vi "dds_host.vi"() -> ()   [LabVIEW 2018]
uses:
  <vilib>/FPGAPlugInAG/PCIe-7841R/niLvFpga_Open_PCIe-7841R.vi
  <vilib>/rvi/interface/common/dynamic/niFpgaDynamicAddResources.vi
  <vilib>/FPGAPlugInAG/Dynamic/niLvFpga_Run_Dynamic.vi
  <vilib>/Utility/error.llb/Error Cluster From Error Code.vi
  <vilib>/rvi/errors/niLvFpgaAdjustHostInterfaceError.vi
  <vilib>/FPGAPlugInAG/Dynamic/niLvFpga_Close_Dynamic.vi
  <vilib>/rvi/interface/nirviOpenFPGA/nirviOpenFPGA.xnode
  FPGA Bitfiles/dds_FPGATarget_ddsfpga_kTR-VUpZgFc.lvbitx
  <vilib>/rvi/interface/nirviMethod/nirviMethod.xnode
  <vilib>/rvi/interface/nirviReadWriteControl/nirviReadWriteControl.xnode
  <vilib>/rvi/interface/nirviCloseFPGA/nirviCloseFPGA.xnode
  <vilib>/rvi/interface/Simulation/niFpgaSimulationCallBeginRW.vi
  NiFpgaLv.dll
  <vilib>/rvi/Analysis/host/Public/NI_FpgaMspHost.lvlib
panel:
  out "slow_freq":dbl
  out "scale factor_slow-dds":fxp<+/-,16,1>
  in  "vpp_slow-dds":dbl
  in  "slow-dds_param":T1={"Sine wave frequency (Hz)"=50.0, "Phase offset (deg)"=0.0} {"Phase offset (deg)" format="%#_6p"; "Sine wave frequency (Hz)" format="%#_6p"}
  in  "z_slow-dds?":bool
  in  "45_sin":bool=TRUE
  in  "23_sin":bool
  in  "01_sin":bool=TRUE
  in  "just x?":bool
  out "synth_settings_client":dbl[](array[numeric])=[8.0, 50000.0]
  out "scale factor 45":fxp<+/-,16,1>=0.20001220703125
  out "scale factor 23":fxp<+/-,16,1>=0.20001220703125
  out "scale factor 01":fxp<+/-,16,1>
  in  "set xy drive network?":bool
  in  "vpp 45":dbl=4.0
  in  "vpp 23":dbl=4.0
  in  "vpp 01":dbl
  in  "Desired loop rate (ticks)":u32=84
  in  "frequency increment":dbl=0.1
  out "requested_freq":dbl(graph)
  out "Sampling Rate\nAchieved?":bool=TRUE
  out "Actual Sample Rate (S/s)":dbl=952380.9523809524 format="%#_6p"
  in  "re-initialize_dds":bool
  in  "fast-dds_param":T1={"Sine wave frequency (Hz)"=50000.0, "Phase offset (deg)"=0.0} {"Phase offset (deg)" format="%#_6p"; "Sine wave frequency (Hz)" format="%#_6p"}
  in  "step_time (ms)":u32=1
  out "error out":errorcluster={"status"=TRUE, "code"=-61169, "source"="sample rate conversion in NI_FpgaMspHost.lvlib:Sample Rate To Loop Time (ticks).vi->dds_host.vi"}
  in  "stop":bool
  # "SINE"
  # "COSINE"
  # "SINE"
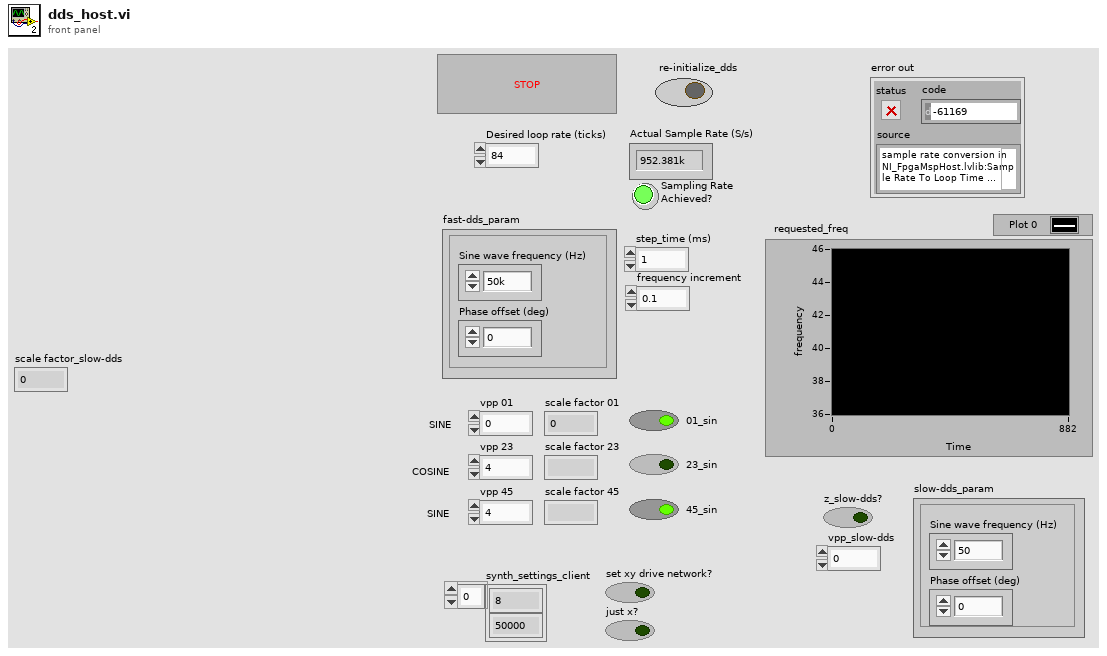
[diagram p1: front panel]
types:
  T1 = cluster{"Sine wave frequency (Hz)":dbl, "Phase offset (deg)":dbl}
  T2 = enum16{"open", "replace", "create", "open or create", "replace or create", "replace or create with confirmation"}
  T3 = cluster{"frequency (periods/tick)":fxp<+,32,0>, "phase offset (periods)":fxp<+,32,0>, fxp<+/-,16,1>, fxp<+,1,1>}
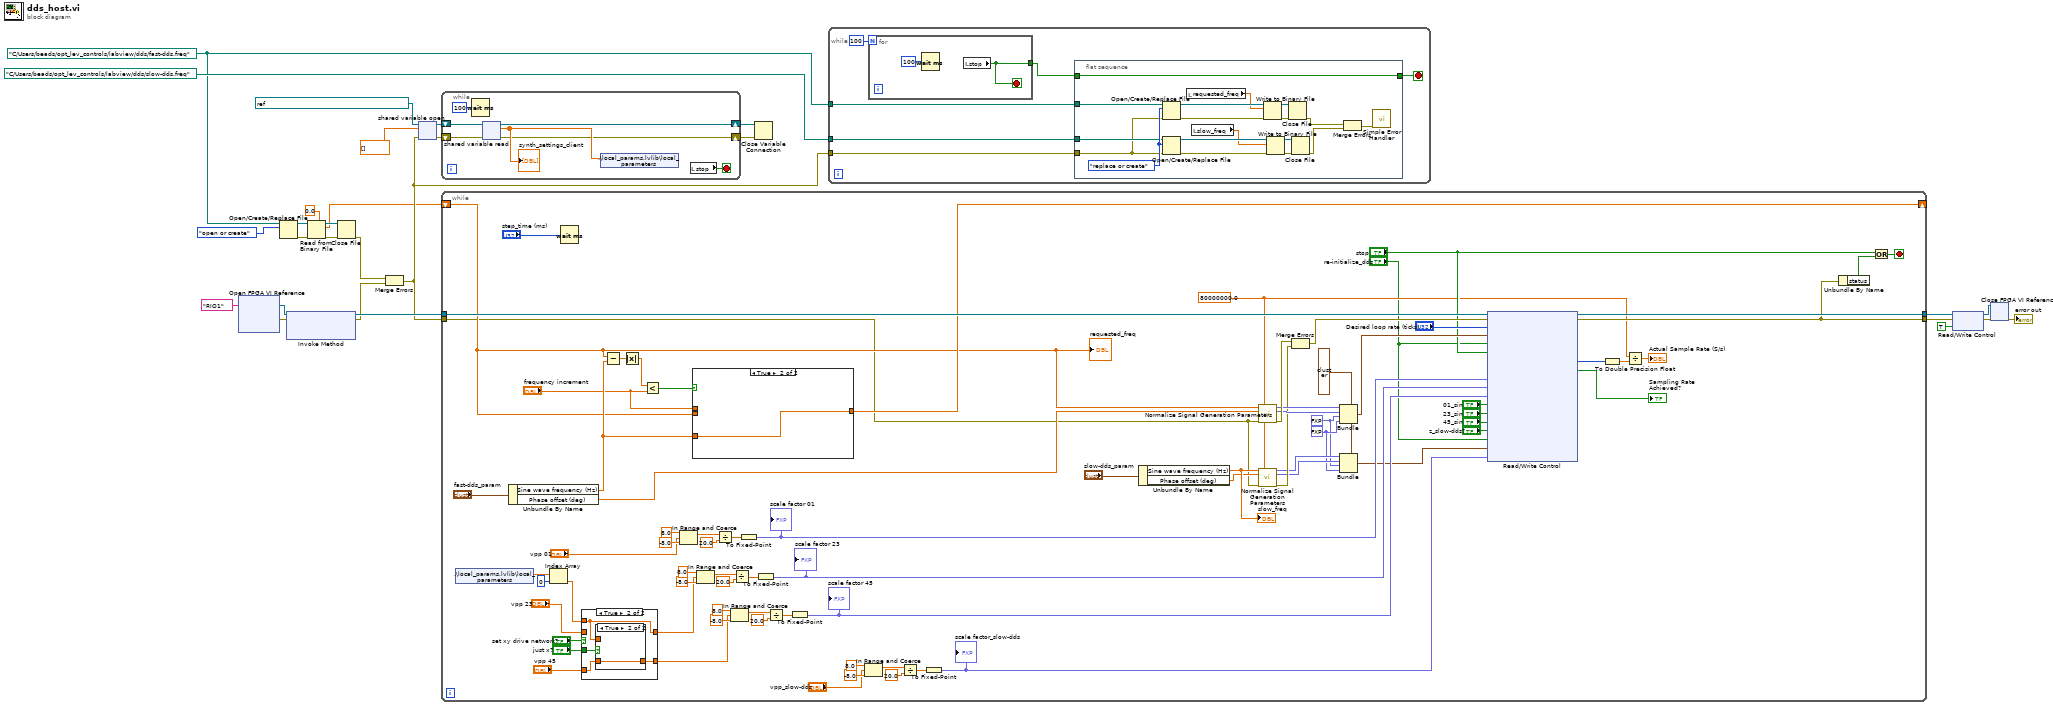
[diagram p0: block diagram]
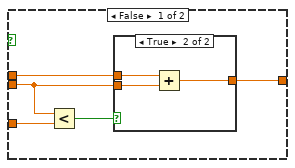
[diagram p4: hidden frame]
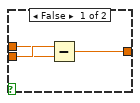
[diagram p5: hidden frame]
diagram:
  w11 = path "C:/Users/beads/opt_lev_controls/labview/dds/fast-dds.freq" ("file path (use dialog)")
  n1 = xnode "Open FPGA VI Reference"("resource name"=tag "RIO1") -> ("FPGA VI Reference Out"=w26:refnum<k20>, "error out"=w27:errorcluster)  [unwired: 1 in]
  n2 = Open/Create/Replace File(file path (use dialog)=w11, operation (0:open)=T2."open or create") -> (refnum out=w9:refnum<file>, error out=w10:errorcluster)  [unwired: 4 in, 1 out]
  n3 = xnode "Invoke Method"("FPGA VI Reference In"=w26, "error in"=w27) -> ("FPGA VI Reference Out"=w25:refnum<k20>, "error out"=w6:errorcluster)  [unwired: 1 in]
  n4 = Read from Binary File(5:0.0, 8:w10, 11:w9) -> (0:w8:errorcluster, 2:w1:dbl, 3:w7:refnum<file>)  [unwired: 3 in, 1 out]
  n5 = Close File(refnum=w7, error in=w8) -> (error out=w5:errorcluster)  [unwired: 1 out]
  n6 = Merge Errors(w5, w6) -> (w2:errorcluster)
  n7 = shared-variable-open(refnum<k21> "ni.var.psp://localhost/daq_lib/synth_settings" ("shared variable refnum in"), w2, dbl[] [] ("synth_settings_client")) -> (w16:refnum<k21>, w15:errorcluster)  [unwired: 1 in]
  n8 = while {
    tunnel: w25 -> [w106]
    tunnel: w2 -> [w44]
    tunnel: [w104] -> w24
    tunnel: [w105] -> w23
    shift-right: [w75] -> _
    shift-left: w1 -> [w74]
    stop <- w102 stop-if-true
    w38 = fxp<+/-,16,1> 0.0
    w42 = T3 {"frequency (periods/tick)"=0.0, "phase offset (periods)"=0.0, 0.0, 0.0} ("cluster")
    w39 = fxp<+,1,1> 0.0
    w45 = 80000000.0 ("FPGA clock rate (Hz)")
    n9 = shared-variable ".\\local_params.lvlib\\local_parameters"() -> (w73:dbl[])  [unwired: 1 in, 1 out]
    n10 = Unbundle By Name("fast-dds_param") -> ("Sine wave frequency (Hz)"=w82:dbl, "Phase offset (deg)"=w88:dbl)
    n11 = Index Array(array=w73, index=0) -> (element=w49:dbl)
    n12 = Wait (ms)(milliseconds to wait="step_time (ms)") -> ()  [unwired: 1 out]
    n13 = case shown="True" "set xy drive network?" {
      tunnel: "vpp 23" -> [w108 _]
      tunnel: [w108 w109] -> w57
      tunnel: "vpp 45" -> [w107 w111]
      tunnel: [w107 w110] -> w50
      tunnel: "just x?" -> [_ w112]
      tunnel: w49 -> [_ w109]
      frame False {
      }
      frame True {
        n14 = case shown="True" w112 {
          tunnel: w111 -> [_ w114]
          tunnel: [w113 w114] -> w110
          tunnel: w109 -> [w113 _]
          frame False {
          }
          frame True {
          }
        }
      }
    }
    n15 = Subtract(x=w74, y=w82) -> (x-y=w84:dbl)
    n16 = Absolute Value(x=w84) -> (abs(x)=w83:dbl)
    n17 = Less?(x=w83, y="frequency increment") -> (x < y?=w80:bool)
    n18 = In Range and Coerce(upper limit=8.0, x="vpp 01", lower limit=-8.0) -> (coerced(x)=w87:dbl)  [unwired: 1 out]
    n19 = case shown="True" w80 {
      tunnel: [w116 w126] -> w75
      tunnel: w74 -> [w115 _]
      tunnel: w82 -> [w119 w126]
      tunnel: "frequency increment" -> [w117 _]
      frame False {
        n20 = Less?(x=w115, y=w119) -> (x < y?=w118:bool)
        n21 = case shown="True" w118 {
          tunnel: w115 -> [w121 w125]
          tunnel: w117 -> [w120 w124]
          tunnel: [w122 w123] -> w116
          frame False {
            n22 = Subtract(x=w121, y=w120) -> (x-y=w122:dbl)
          }
          frame True {
            n23 = Add(x=w124, y=w125) -> (x+y=w123:dbl)
          }
        }
      }
      frame True {
      }
    }
    n24 = In Range and Coerce(upper limit=8.0, x=w57, lower limit=-8.0) -> (coerced(x)=w61:dbl)  [unwired: 1 out]
    n25 = Divide(x=w87, y=20.0) -> (x/y=w94:dbl)
    n26 = In Range and Coerce(upper limit=8.0, x=w50, lower limit=-8.0) -> (coerced(x)=w54:dbl)  [unwired: 1 out]
    n27 = Divide(x=w61, y=20.0) -> (x/y=w62:dbl)
    n28 = To Fixed-Point(number=w94) -> (fixed-point=w78:fxp<+/-,16,1>)  [unwired: 1 in]
    "scale factor 01" <- w78
    n29 = To Fixed-Point(number=w62) -> (fixed-point=w58:fxp<+/-,16,1>)  [unwired: 1 in]
    "scale factor 23" <- w58
    n30 = Divide(x=w54, y=20.0) -> (x/y=w55:dbl)
    n31 = To Fixed-Point(number=w55) -> (fixed-point=w51:fxp<+/-,16,1>)  [unwired: 1 in]
    "scale factor 45" <- w51
    n32 = In Range and Coerce(upper limit=8.0, x="vpp_slow-dds", lower limit=-8.0) -> (coerced(x)=w34:dbl)  [unwired: 1 out]
    n33 = Divide(x=w34, y=20.0) -> (x/y=w35:dbl)
    n34 = To Fixed-Point(number=w35) -> (fixed-point=w30:fxp<+/-,16,1>)  [unwired: 1 in]
    "scale factor_slow-dds" <- w30
    n35 = Unbundle By Name("slow-dds_param") -> ("Sine wave frequency (Hz)"=w47:dbl, "Phase offset (deg)"=w46:dbl)
    "slow_freq" <- w47
    n36 = call <vilib>:"Normalize Signal Generation Parameters.vi"("frequency (Hz)"=w74, "FPGA clock rate (Hz)"=w45, "phase offset (deg)"=w88, "error in (no error)"=w44) -> ("frequency (periods/tick)"=w97:fxp<+,32,0>, "phase offset (periods)"=w96:fxp<+,32,0>, "error out"=w99:errorcluster)  [unwired: 6 in, 3 out]
    n37 = call <vilib>:"Normalize Signal Generation Parameters.vi"("frequency (Hz)"=w47, "FPGA clock rate (Hz)"=w45, "phase offset (deg)"=w46, "error in (no error)"=w44) -> ("frequency (periods/tick)"=w41:fxp<+,32,0>, "phase offset (periods)"=w40:fxp<+,32,0>, "error out"=w43:errorcluster)  [unwired: 6 in, 3 out]
    n38 = Merge Errors(w99, w43) -> (w98:errorcluster)
    n39 = Bundle(cluster=w42, "frequency (periods/tick)"=w97, "phase offset (periods)"=w96, w38, w39) -> (w93:T3)
    n40 = Bundle(cluster=w42, "frequency (periods/tick)"=w41, "phase offset (periods)"=w40, w38, w39) -> (w37:T3)
    n41 = xnode "Read/Write Control"("FPGA VI Reference In"=w106, "error in"=w98, "Desired loop rate (ticks)"="Desired loop rate (ticks)", "sinewave-props_fast-dds"=w93, "Initialize fast-dds"="re-initialize_dds", "stop"="stop", "fast-dds_scale01"=w78, "fast-dds_scale23"=w58, "fast-dds_scale45"=w51, "01_sin"="01_sin", "23_sin"="23_sin", "45_sin"="45_sin", "z_slow-dds?"="z_slow-dds?", "Initialize slow-dds"="re-initialize_dds", "sinewave-props_slow-dds"=w37, "slow-dds_scale"=w30) -> ("FPGA VI Reference Out"=w105:refnum<k20>, "error out"=w104:errorcluster, "Actual loop rate"=w90:u32, "Sampling rate achieved?"=→"Sampling Rate\nAchieved?":bool)
    n42 = To Double Precision Float(number=w90) -> (double precision float=w92:dbl)
    n43 = Divide(x=w45, y=w92) -> (x/y=→"Actual Sample Rate (S/s)":dbl)
    n44 = Unbundle By Name(w104) -> ("status"=w103:bool)
    n45 = Or(x="stop", y=w103) -> (x .or. y?=w102:bool)
    "requested_freq" <- w74
  }
  n46 = while {
    shift-right: [w128] -> w14
    shift-left: w16 -> [w131]
    shift-right: [w127] -> w13
    shift-left: w15 -> [w130]
    stop <- w132 stop-if-true
    n47 = Wait (ms)(milliseconds to wait=u32 100) -> ()  [unwired: 1 out]
    n48 = shared-variable-read(w131, w130) -> (w128:refnum<k21>, w127:errorcluster, w129:dbl[])  [unwired: 1 out]
    "synth_settings_client" <- w129
    n49 = shared-variable ".\\local_params.lvlib\\local_parameters"(w129) -> ()  [unwired: 1 in, 1 out]
    n50 = local read "stop"() -> (w132:bool)
  }
  n51 = Close Variable Connection(8:w13, 11:w14) -> ()  [unwired: 1 out]
  n52 = while {
    tunnel: w11 -> [w139]
    tunnel: path "C:/Users/beads/opt_lev_controls/labview/dds/slow-dds.freq" ("file path (use dialog)") -> [w138]
    tunnel: w2 -> [w136]
    stop <- w134 stop-if-true
    n53 = for {
      N: 100 -> [_]
      tunnel: [w159] -> w135
      stop <- w159 stop-if-true
      n54 = Wait (ms)(milliseconds to wait=u32 100) -> ()  [unwired: 1 out]
      n55 = local read "stop"() -> (w159:bool)
    }
    n56 = flat-sequence {
      tunnel: w139 -> [w143]
      tunnel: w138 -> [w142]
      tunnel: w136 -> [w141]
      tunnel: w135 -> [w140]
      tunnel: [w140] -> w134
      frame #0 {
        w157 = T2."replace or create" ("operation (0:open)")
        n57 = Open/Create/Replace File(file path (use dialog)=w142, error in=w141, operation (0:open)=w157) -> (refnum out=w152:refnum<file>, error out=w153:errorcluster)  [unwired: 3 in, 1 out]
        n58 = Open/Create/Replace File(file path (use dialog)=w143, error in=w141, operation (0:open)=w157) -> (refnum out=w156:refnum<file>, error out=w155:errorcluster)  [unwired: 3 in, 1 out]
        n59 = local read "requested_freq"() -> (w154:dbl)
        n60 = local read "slow_freq"() -> (w151:dbl)
        n61 = Write to Binary File(file (use dialog)=w156, data=w154, error in=w155) -> (refnum out=w149:refnum<file>, error out=w150:errorcluster)  [unwired: 3 in, 1 out]
        n62 = Write to Binary File(file (use dialog)=w152, data=w151, error in=w153) -> (refnum out=w148:refnum<file>, error out=w147:errorcluster)  [unwired: 3 in, 1 out]
        n63 = Close File(refnum=w149, error in=w150) -> (error out=w146:errorcluster)  [unwired: 1 out]
        n64 = Close File(refnum=w148, error in=w147) -> (error out=w145:errorcluster)  [unwired: 1 out]
        n65 = Merge Errors(w146, w145) -> (w144:errorcluster)
        n66 = call <vilib>:"Simple Error Handler.vi"("error in (no error)"=w144) -> ()  [unwired: 4 in, 5 out]
      }
    }
  }
  n67 = xnode "Read/Write Control"("FPGA VI Reference In"=w23, "error in"=w24, "stop"=TRUE) -> ("FPGA VI Reference Out"=w22:refnum<k20>, "error out"=w21:errorcluster)
  n68 = xnode "Close FPGA VI Reference"("FPGA VI Reference In"=w22, "error in"=w21) -> ("error out"=→"error out":errorcluster)
